vi "CheckImage.vi"(7 "Score cutoff":dbl, 8 "error in":errorcluster, 9 "Color Components":T3={"Hue"={110.0, 142.0}, "Sat"={138.0, 255.0}, "Val"={139.0, 198.0}} {"Val" scale=0.0..255.0; "Sat" scale=0.0..255.0; "Hue" scale=0.0..255.0 scale format="%#_3g"}, 10 "Color System":u16(ring)=2 items=["RGB", "HSL", "HSV", "HSI"], 11 "Image":T2) -> (0 "error out":errorcluster, 1 "Hot?":bool, 3 "Image out":T2)   [LabVIEW 2015]
doc: "Determines if the goal is hot or not and returns a boolean to indicate this. Does not calculate the image to the target."
uses:
  <vilib>/vision/Image Controls.llb/IMAQ Image.ctl
  Example_Code/2014 Target Detection/TargetType.ctl
panel:
  out "Scores.State":T1
  in  "Area Size Limit %":dbl=0.06 format="%#_13g"
  out "Mask":T2(plugin-control)
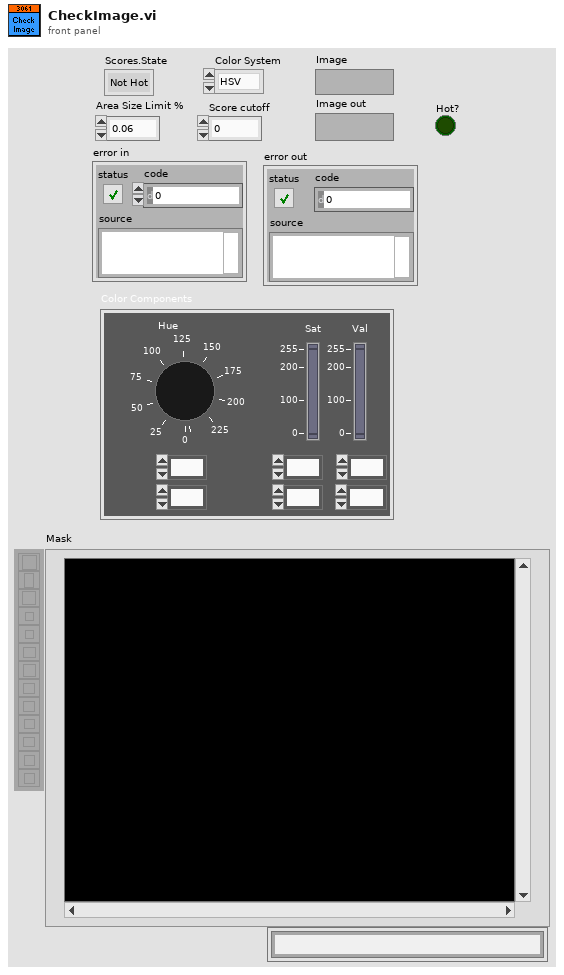
[diagram p1: front panel]
types:
  T1 = typedef "TargetType.ctl" = enum16{"Not Hot", "Hot"}
  T2 = typedef "IMAQ Image.ctl" = refnum<image>
  T3 = cluster{"Hue":cluster{dbl, dbl}, "Sat":cluster{dbl, dbl}, "Val":cluster{dbl, dbl}}
  T4 = cluster{"Horizontal":bool, "Aspect Score":dbl, "Rect Score":dbl, cluster{"Left":dbl, "Top":dbl, "Right":dbl, "Bottom":dbl}, "Equiv H":dbl, "Equiv V":dbl}[]
  T5 = cluster{"Scores":cluster{"Total":dbl, "Left":dbl, "Right":dbl, "Ratio":dbl, "Vertical":dbl, "index":i32, "State":T1}, "Verticals":cluster{"Horizontal?":bool, "Aspect Score":dbl, "Rect Score":dbl, cluster{"Left":dbl, "Top":dbl, "Right":dbl, "Bottom":dbl}, "Equiv H":dbl, "Equiv V":dbl}, "Horizontals":cluster{"Horizontal?":bool, "Aspect Score":dbl, "Rect Score":dbl, cluster{"Left":dbl, "Top":dbl, "Right":dbl, "Bottom":dbl}, "Equiv H":dbl, "Equiv V":dbl}, "Validated":bool}[]
  T6 = cluster{"Scores":cluster{"Total":dbl, "Left":dbl, "Right":dbl, "Ratio":dbl, "Vertical":dbl, "index":i32, "State":T1}, "Verticals":cluster{"Horizontal?":bool, "Aspect Score":dbl, "Rect Score":dbl, cluster{"Left":dbl, "Top":dbl, "Right":dbl, "Bottom":dbl}, "Equiv H":dbl, "Equiv V":dbl}, "Horizontals":cluster{"Horizontal?":bool, "Aspect Score":dbl, "Rect Score":dbl, cluster{"Left":dbl, "Top":dbl, "Right":dbl, "Bottom":dbl}, "Equiv H":dbl, "Equiv V":dbl}, "Validated":bool}
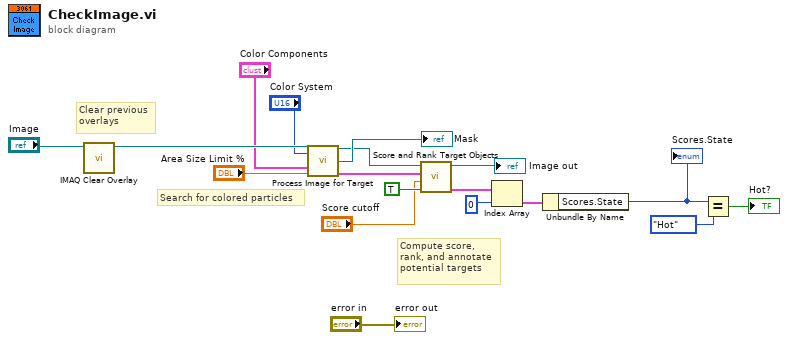
[diagram p0: block diagram]
diagram:
  # "Clear previous\noverlays"
  # "Search for colored particles"
  # "Compute score,\nrank, and annotate\npotential targets"
  n1 = call "IMAQ Clear Overlay"("Image"="Image") -> ("Image Out"=w14:T2)  [unwired: 9 in, 1 out]
  n2 = call "Process Image for Target.vi"("Src Image"=w14, "Color Mode"="Color System", "Color Components"="Color Components", "Area Cutoff %"="Area Size Limit %") -> ("Src Image Out"=w16:T2, "Threshold"=→"Mask":T2, "Particles"=w15:T4)  [unwired: 9 in]
  n3 = call "Score and Rank Target Objects.vi"("Annotate"=TRUE, "Score Limit"="Score cutoff", "Particles"=w15, "Image in"=w16) -> ("Target Info"=w4:T5, "Annotated Image"=→"Image out":T2)  [unwired: 6 in]
  n4 = Index Array(array=w4, index=0) -> (element=w8:T6)
  n5 = Unbundle By Name(w8) -> ("Scores.State"=w3:T1)
  "Scores.State" <- w3
  n6 = Equal?(x=w3, y=TargetType."Hot") -> (x = y?=→"Hot?":bool)
  "error out" <- "error in"
